vi "DriveForDistance.vi"() -> ()   [LabVIEW 2020]
uses:
  Framework/Robot Global Data.vi
panel:
  in  "NoWait":bool
  in  "Distance":dbl
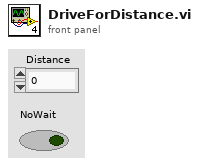
[diagram p1: front panel]
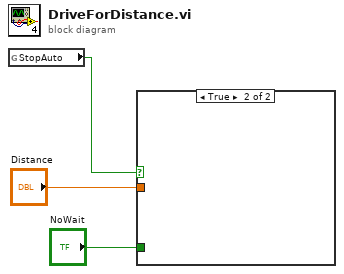
[diagram p0: block diagram]
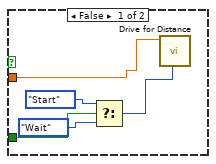
[diagram p2: hidden frame]
diagram:
  n1 = global read "Robot Global Data.vi" "StopAuto"() -> (w3:bool)
  n2 = case shown="True" w3 {
    tunnel: "NoWait" -> [w7 _]
    tunnel: "Distance" -> [w5 _]
    frame False {
      n3 = Select(t=enum16{"Start", "Wait"}."Start" ("Synchronization"), s=w7, f=enum16{"Start", "Wait"}."Wait" ("Synchronization")) -> (s? t:f=w4:enum16{"Start", "Wait"})
      n4 = call "Drive for Distance.vi"("Synchronication"=w4, "Distance"=w5) -> ()  [unwired: 9 in, 1 out]
    }
    frame True {
    }
  }
